vi "niRFUtil FTW Generate VBW Response.vi"(1 "Minimum Selectivity (dB)":dbl=70.0 format="%.2f", 2 "df (Hz)":dbl format="%^.2e", 3 "VBW (Hz)":dbl format="%^.2e", 4 "Center Frequency (Hz)":dbl format="%^.6e") -> (0 "Filter Power Response":T1 {"y" min=0 max=127 format="%.2f"; "dx" format="%^.2e"; "x0" format="%^.2e"})   [LabVIEW 2015, in "niRFUtil.lvlib"]
doc: "(c) Copyright 2006, National Instruments, Inc. This VI may not be duplicated, sold, or distributed without written consent from National Instruments."
uses:
  niRFUtil.lvlib
  Includes/niRFUtil INC Real Waveform.ctl
  Includes/niRFUtil INC Real Array.ctl
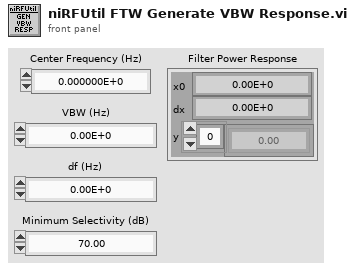
[diagram p1: front panel]
types:
  T1 = typedef "niRFUtil.lvlib/niRFUtil INC Real Waveform.ctl" = cluster{"x0":dbl, "dx":dbl, "y":T2}
  T2 = typedef "niRFUtil.lvlib/niRFUtil INC Real Array.ctl" = sgl[]
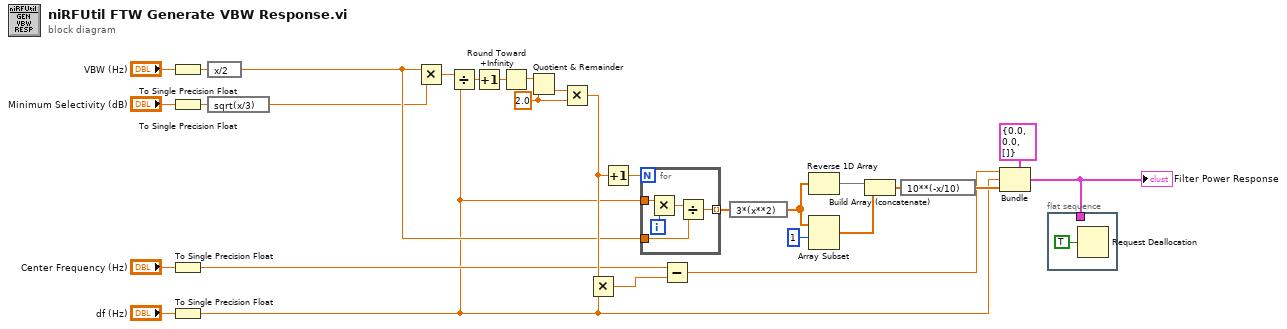
[diagram p0: block diagram]
diagram:
  w21 = 2.0 ("y")
  n1 = To Single Precision Float(number="VBW (Hz)") -> (single precision float=w7:sgl)
  n2 = To Single Precision Float(number="Minimum Selectivity (dB)") -> (single precision float=w5:sgl)
  n3 = To Single Precision Float(number="Center Frequency (Hz)") -> (single precision float=w3:sgl)
  n4 = To Single Precision Float(number="df (Hz)") -> (single precision float=w1:sgl)
  n5 = expression code="x/2"(w7) -> (w13:sgl)
  n6 = expression code="sqrt(x/3)"(w5) -> (w12:sgl)
  n7 = Multiply(x=w13, y=w12) -> (x*y=w29:sgl)
  n8 = Divide(x=w29, y=w1) -> (x/y=w24:sgl)
  n9 = Increment(x=w24) -> (x+1=w19:sgl)
  n10 = Round Toward +Infinity(x=w19) -> (ceil(x): smallest int >= x=w23:sgl)
  n11 = Quotient & Remainder(x=w23, y=w21) -> (floor(x/y)=w22:dbl)  [unwired: 1 out]
  n12 = Multiply(x=w22, y=w21) -> (x*y=w20:dbl)
  n13 = Multiply(x=w20, y=w1) -> (x*y=w26:dbl)
  n14 = Increment(x=w20) -> (x+1=w27:dbl)
  n15 = for {
    N: w27 -> [_]
    tunnel: w1 -> [w34]
    tunnel: w13 -> [w31]
    tunnel: [w30] -> w11 mode=indexing
    i -> [w33]
    n16 = Multiply(x=w34, y=w33) -> (x*y=w32:sgl)
    n17 = Divide(x=w32, y=w31) -> (x/y=w30:sgl)
  }
  n18 = Subtract(x=w3, y=w26) -> (x-y=w14:dbl)
  n19 = expression code="3*(x**2)"(w11) -> (w25:sgl[])
  n20 = Reverse 1D Array(array=w25) -> (reversed array=w17:sgl[])
  n21 = Array Subset(array=w25, index=1) -> (w16:sgl[])  [unwired: 1 in]
  n22 = Build Array (concatenate)(w17, w16) -> (w15:sgl[])
  n23 = expression code="10**(-x/10)"(w15) -> (w18:sgl[])
  n24 = Bundle(cluster=T1 {"x0"=0.0, "dx"=0.0, "y"=[]} ("Filter"), "x0"=w14, "dx"=w1, "y"=w18) -> (w9:T1)
  "Filter Power Response" <- w9
  n25 = flat-sequence {
    tunnel: w9 -> [_]
    frame #0 {
      n26 = Request Deallocation(TRUE ("flag")) -> ()
    }
  }
